vi "Align VI windows.vi"(4 "Keep on screen [T]":bool=TRUE, 5 "Align to":enum16{"FP", "BD"}(ring), 6 "Offset":cluster{"X":dbl, "Y":dbl}, 7 "Position [Center]":T2(ring)=enum."Center", 8 "error in":errorcluster, 10 "VI to Move Ref":refnum<vi>, 11 "Stationary VI Ref":refnum<vi>) -> (0 "error out":errorcluster)   [LabVIEW 2023]
doc: "Align two VI windows to center or one of the calling VIs corners. Offset is from calling VIs top left corner. \n\nYou can align to the stationary VI's front panel (default) or block diagram.\n\nWindow alignment can be on center or 12 other possible positions.\n\nThis VI operates on input error (input err merged with output error).\n\n'Keep on screen' (default=T) will automatically offset VI to Move window position to keep the top-left corner on the current monitor, to ensure that the title bar can be grabbed for moving the window."
uses:
  <userlib>/_OpenG.lib/appcontrol/appcontrol.llb/openg_application_control.lvlib
panel:
  out "New VI bounds":T1
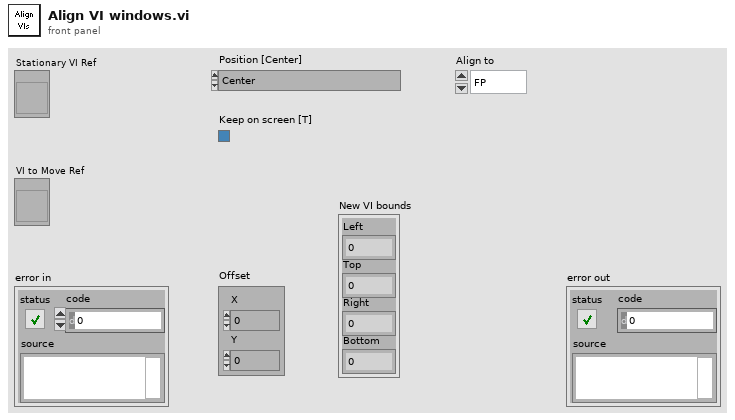
[diagram p1: front panel]
types:
  T1 = cluster{"Left":i16, "Top":i16, "Right":i16, "Bottom":i16}
  T2 = enum16{"Top Left", "Bottom Left", "Top Right", "Bottom Right", "Center", "Above Left", "Above Right", "Below Left", "Below Right", "Left Bottom", "Left Top", "Right Bottom", "Right Top", "Outside TL Corner", "Outside TR Corner", "Outside BL Corner", "Outside BR Corner"}
  T3 = enum16{"Top Left", "Bottom Left", "Top Right", "Bottom Right", "Center"}
  T4 = typedef "LVRectTypeDef.ctl" = cluster{"Left":i16, "Top":i16, "Right":i16, "Bottom":i16}
  T5 = typedef "x,y cluster_DBL.ctl" = cluster{"X":dbl, "Y":dbl}
  T6 = cluster{"left":i16, "top":i16, "right":i16, "bottom":i16}
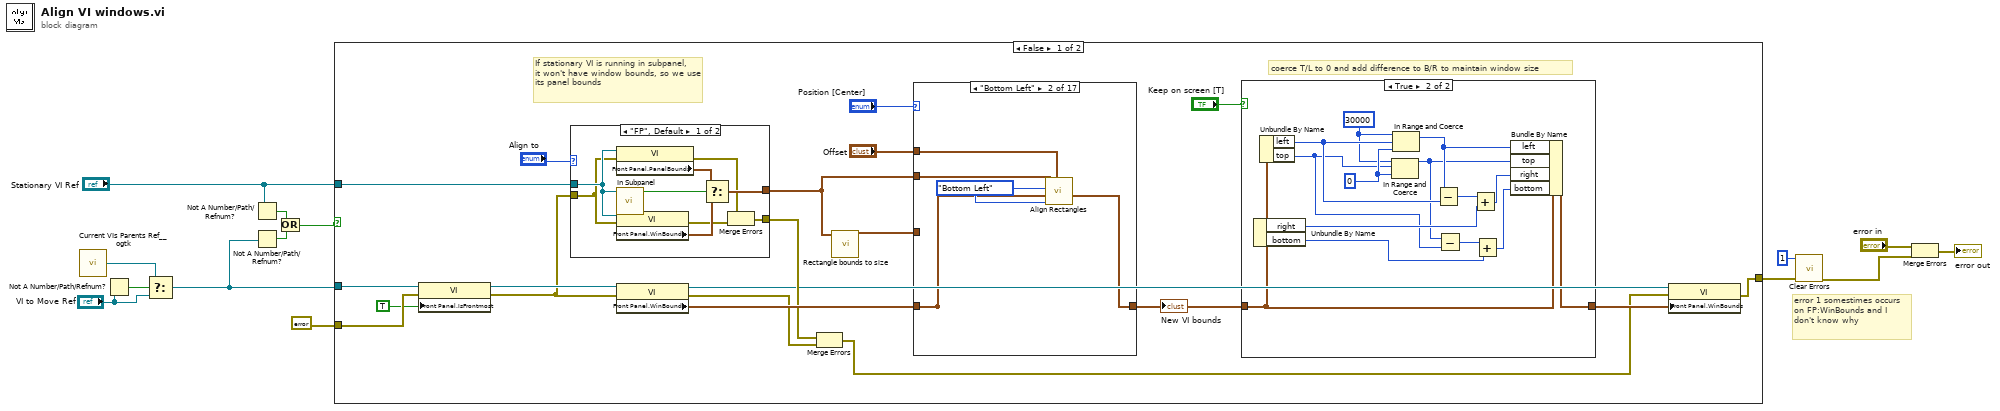
[diagram p0: block diagram]
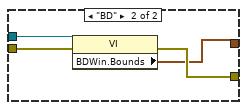
[diagram p3: hidden frame]
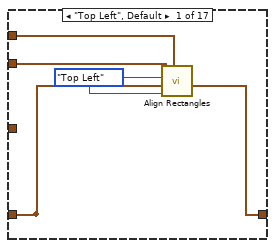
[diagram p4: hidden frame]
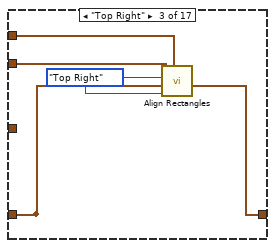
[diagram p5: hidden frame]
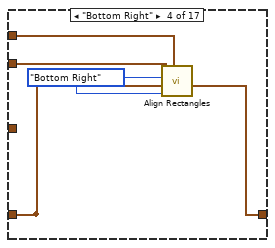
[diagram p6: hidden frame]
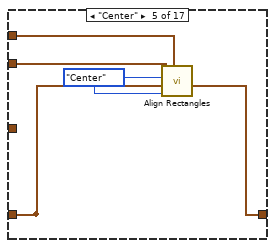
[diagram p7: hidden frame]
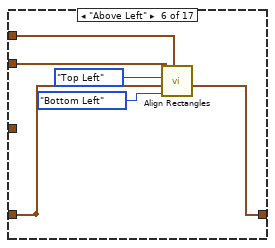
[diagram p8: hidden frame]
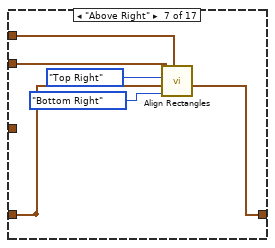
[diagram p9: hidden frame]
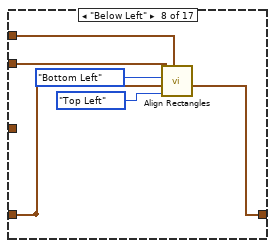
[diagram p10: hidden frame]
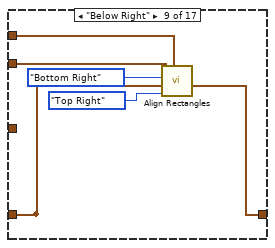
[diagram p11: hidden frame]
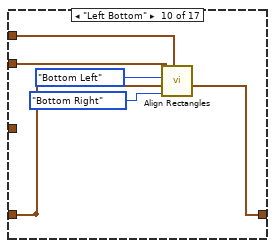
[diagram p12: hidden frame]
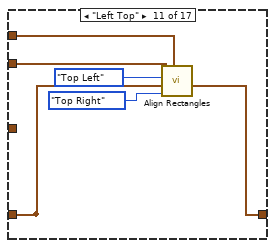
[diagram p13: hidden frame]
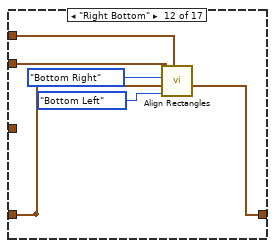
[diagram p14: hidden frame]
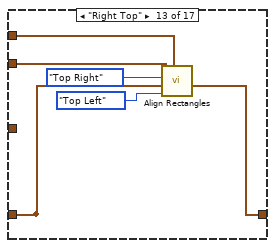
[diagram p15: hidden frame]
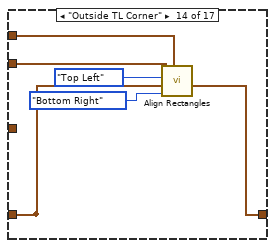
[diagram p16: hidden frame]
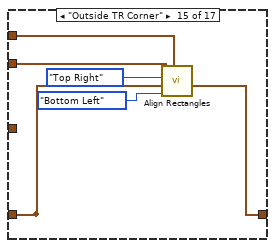
[diagram p17: hidden frame]
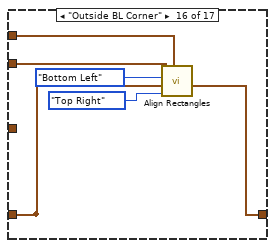
[diagram p18: hidden frame]
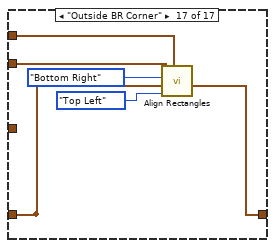
[diagram p19: hidden frame]
diagram:
  # "error 1 somestimes occurs on FP:WinBounds and I don't know why"
  n1 = call <userlib>:"Current VIs Parents Ref__ogtk.vi"() -> ("Calling VI's Reference"=w1:refnum<vi>)  [unwired: 2 in]
  n2 = Not A Number/Path/Refnum?(number/path/refnum="VI to Move Ref") -> (NaN/Path/Refnum?=w4:bool)
  n3 = Select(t=w1, s=w4, f="VI to Move Ref") -> (s? t:f=w2:refnum<vi>)
  n4 = Not A Number/Path/Refnum?(number/path/refnum="Stationary VI Ref") -> (NaN/Path/Refnum?=w14:bool)
  n5 = Not A Number/Path/Refnum?(number/path/refnum=w2) -> (NaN/Path/Refnum?=w13:bool)
  n6 = Or(x=w14, y=w13) -> (x .or. y?=w11:bool)
  n7 = case shown="False" w11 {
    tunnel: "Stationary VI Ref" -> [w29 _]
    tunnel: errorcluster {"status"=FALSE, "code"=0, "source"=""} ("error in (no error)") -> [w16 w159]
    tunnel: [w30 w159] -> w7
    tunnel: w2 -> [w19 _]
    frame False {
      # "coerce T/L to 0 and add difference to B/R to maintain window size"
      # "If stationary VI is running in subpanel, it won't have window bounds, so we use its panel bounds"
      n8 = property class="VI"(reference=w19, error in=w16, "Front Panel.IsFrontmost"=TRUE ("Front Panel Window:Is Frontmost")) -> (reference out=w18:refnum<vi>, error out=w17:errorcluster)
      n9 = case shown="\"FP\", Default" "Align to" {
        tunnel: w29 -> [w57 w61]
        tunnel: [w54 w58] -> w28
        tunnel: w17 -> [w53 w60]
        tunnel: [w50 w59] -> w26
        frame "FP", Default {
          n10 = property class="VI"(reference=w57, error in=w53) -> (error out=w51:errorcluster, "Front Panel.PanelBounds"=w56:T4)  [unwired: 1 out]
          n11 = call "In Subpanel.vi"("VI Ref"=w57) -> ("VI in SubPanel?"=w49:bool)  [unwired: 10 in]
          n12 = property class="VI"(reference=w57, error in=w53) -> (error out=w52:errorcluster, "Front Panel.WinBounds"=w55:T4)  [unwired: 1 out]
          n13 = Select(t=w56, s=w49, f=w55) -> (s? t:f=w54:T4)
          n14 = Merge Errors(w51, w52) -> (w50:errorcluster)
        }
        frame "BD" {
          n15 = property class="VI"(reference=w61, error in=w60) -> (error out=w59:errorcluster, "BDWin.Bounds"=w58:T4)  [unwired: 1 out]
        }
      }
      n16 = property class="VI"(reference=w18, error in=w17) -> (error out=w21:errorcluster, "Front Panel.WinBounds"=w27:T4)  [unwired: 1 out]
      n17 = Merge Errors(w26, w21) -> (w20:errorcluster)
      n18 = call "Rectangle bounds to size.vi"("bounds"=w28) -> ("size"=w32:T5)  [unwired: 6 in, 4 out]
      n19 = case shown="\"Bottom Left\"" "Position [Center]" {
        tunnel: w32 -> [_ _ _ _ _ _ _ _ _ _ _ _ _ _ _ _ _]
        tunnel: w28 -> [w63 w68 w73 w78 w83 w89 w95 w101 w107 w113 w119 w125 w131 w137 w143 w149 w155]
        tunnel: [w62 w67 w72 w77 w82 w88 w94 w100 w106 w112 w118 w124 w130 w136 w142 w148 w154] -> _
        tunnel: "Offset" -> [w65 w70 w75 w80 w85 w91 w97 w103 w109 w115 w121 w127 w133 w139 w145 w151 w157]
        tunnel: [w64 w69 w74 w79 w84 w90 w96 w102 w108 w114 w120 w126 w132 w138 w144 w150 w156] -> w24
        tunnel: w27 -> [w62 w67 w72 w77 w82 w88 w94 w100 w106 w112 w118 w124 w130 w136 w142 w148 w154]
        frame "Top Left", Default {
          w66 = T3."Top Left" ("Position 1 [Top-Left]")
          n20 = call "Align Rectangles.vi"("Offset"=w65, "Position 2 [Top-Left]"=w66, "rect 2"=w62, "Position 1 [Top-Left]"=w66, "rect 1"=w63) -> ("rect out"=w64:T6)  [unwired: 6 in]
        }
        frame "Bottom Left" {
          w71 = T3."Bottom Left" ("Position 1 [Top-Left]")
          n21 = call "Align Rectangles.vi"("Offset"=w70, "Position 2 [Top-Left]"=w71, "rect 2"=w67, "Position 1 [Top-Left]"=w71, "rect 1"=w68) -> ("rect out"=w69:T6)  [unwired: 6 in]
        }
        frame "Top Right" {
          w76 = T3."Top Right" ("Position 1 [Top-Left]")
          n22 = call "Align Rectangles.vi"("Offset"=w75, "Position 2 [Top-Left]"=w76, "rect 2"=w72, "Position 1 [Top-Left]"=w76, "rect 1"=w73) -> ("rect out"=w74:T6)  [unwired: 6 in]
        }
        frame "Bottom Right" {
          w81 = T3."Bottom Right" ("Position 1 [Top-Left]")
          n23 = call "Align Rectangles.vi"("Offset"=w80, "Position 2 [Top-Left]"=w81, "rect 2"=w77, "Position 1 [Top-Left]"=w81, "rect 1"=w78) -> ("rect out"=w79:T6)  [unwired: 6 in]
        }
        frame "Center" {
          w86 = T3."Center" ("Position 1 [Top-Left]")
          n24 = call "Align Rectangles.vi"("Offset"=w85, "Position 2 [Top-Left]"=w86, "rect 2"=w82, "Position 1 [Top-Left]"=w86, "rect 1"=w83) -> ("rect out"=w84:T6)  [unwired: 6 in]
        }
        frame "Above Left" {
          n25 = call "Align Rectangles.vi"("Offset"=w91, "Position 2 [Top-Left]"=T3."Bottom Left" ("Position 1 [Top-Left]"), "rect 2"=w88, "Position 1 [Top-Left]"=T3."Top Left", "rect 1"=w89) -> ("rect out"=w90:T6)  [unwired: 6 in]
        }
        frame "Above Right" {
          n26 = call "Align Rectangles.vi"("Offset"=w97, "Position 2 [Top-Left]"=T3."Bottom Right" ("Position 1 [Top-Left]"), "rect 2"=w94, "Position 1 [Top-Left]"=T3."Top Right", "rect 1"=w95) -> ("rect out"=w96:T6)  [unwired: 6 in]
        }
        frame "Below Left" {
          n27 = call "Align Rectangles.vi"("Offset"=w103, "Position 2 [Top-Left]"=T3."Top Left" ("Position 1 [Top-Left]"), "rect 2"=w100, "Position 1 [Top-Left]"=T3."Bottom Left", "rect 1"=w101) -> ("rect out"=w102:T6)  [unwired: 6 in]
        }
        frame "Below Right" {
          n28 = call "Align Rectangles.vi"("Offset"=w109, "Position 2 [Top-Left]"=T3."Top Right" ("Position 1 [Top-Left]"), "rect 2"=w106, "Position 1 [Top-Left]"=T3."Bottom Right", "rect 1"=w107) -> ("rect out"=w108:T6)  [unwired: 6 in]
        }
        frame "Left Bottom" {
          n29 = call "Align Rectangles.vi"("Offset"=w115, "Position 2 [Top-Left]"=T3."Bottom Right" ("Position 1 [Top-Left]"), "rect 2"=w112, "Position 1 [Top-Left]"=T3."Bottom Left", "rect 1"=w113) -> ("rect out"=w114:T6)  [unwired: 6 in]
        }
        frame "Left Top" {
          n30 = call "Align Rectangles.vi"("Offset"=w121, "Position 2 [Top-Left]"=T3."Top Right" ("Position 1 [Top-Left]"), "rect 2"=w118, "Position 1 [Top-Left]"=T3."Top Left", "rect 1"=w119) -> ("rect out"=w120:T6)  [unwired: 6 in]
        }
        frame "Right Bottom" {
          n31 = call "Align Rectangles.vi"("Offset"=w127, "Position 2 [Top-Left]"=T3."Bottom Left" ("Position 1 [Top-Left]"), "rect 2"=w124, "Position 1 [Top-Left]"=T3."Bottom Right", "rect 1"=w125) -> ("rect out"=w126:T6)  [unwired: 6 in]
        }
        frame "Right Top" {
          n32 = call "Align Rectangles.vi"("Offset"=w133, "Position 2 [Top-Left]"=T3."Top Left" ("Position 1 [Top-Left]"), "rect 2"=w130, "Position 1 [Top-Left]"=T3."Top Right", "rect 1"=w131) -> ("rect out"=w132:T6)  [unwired: 6 in]
        }
        frame "Outside TL Corner" {
          n33 = call "Align Rectangles.vi"("Offset"=w139, "Position 2 [Top-Left]"=T3."Bottom Right" ("Position 1 [Top-Left]"), "rect 2"=w136, "Position 1 [Top-Left]"=T3."Top Left", "rect 1"=w137) -> ("rect out"=w138:T6)  [unwired: 6 in]
        }
        frame "Outside TR Corner" {
          n34 = call "Align Rectangles.vi"("Offset"=w145, "Position 2 [Top-Left]"=T3."Bottom Left" ("Position 1 [Top-Left]"), "rect 2"=w142, "Position 1 [Top-Left]"=T3."Top Right", "rect 1"=w143) -> ("rect out"=w144:T6)  [unwired: 6 in]
        }
        frame "Outside BL Corner" {
          n35 = call "Align Rectangles.vi"("Offset"=w151, "Position 2 [Top-Left]"=T3."Top Right" ("Position 1 [Top-Left]"), "rect 2"=w148, "Position 1 [Top-Left]"=T3."Bottom Left", "rect 1"=w149) -> ("rect out"=w150:T6)  [unwired: 6 in]
        }
        frame "Outside BR Corner" {
          n36 = call "Align Rectangles.vi"("Offset"=w157, "Position 2 [Top-Left]"=T3."Top Left" ("Position 1 [Top-Left]"), "rect 2"=w154, "Position 1 [Top-Left]"=T3."Bottom Right", "rect 1"=w155) -> ("rect out"=w156:T6)  [unwired: 6 in]
        }
      }
      "New VI bounds" <- w24
      n37 = case shown="True" "Keep on screen [T]" {
        tunnel: w24 -> [w34 w44]
        tunnel: [w34 w47] -> w22
        frame False {
        }
        frame True {
          w35 = 30000 ("upper limit")
          w48 = 0
          n38 = Unbundle By Name(w44) -> ("right"=w42:i16, "bottom"=w36:i16)
          n39 = Unbundle By Name(w44) -> ("left"=w45:i16, "top"=w37:i16)
          n40 = In Range and Coerce(upper limit=w35, x=w37, lower limit=w48) -> (coerced(x)=w39:i32)  [unwired: 1 out]
          n41 = In Range and Coerce(upper limit=w35, x=w45, lower limit=w48) -> (coerced(x)=w46:i32)  [unwired: 1 out]
          n42 = Subtract(x=w46, y=w45) -> (x-y=w43:i32)
          n43 = Subtract(x=w39, y=w37) -> (x-y=w40:i32)
          n44 = Add(x=w43, y=w42) -> (x+y=w41:i32)
          n45 = Add(x=w40, y=w36) -> (x+y=w38:i32)
          n46 = Bundle By Name(cluster=w44, "left"=w46, "top"=w39, "right"=w41, "bottom"=w38) -> (w47:T6)
        }
      }
      n47 = property class="VI"(reference=w18, error in=w20, "Front Panel.WinBounds"=w22) -> (error out=w30:errorcluster)  [unwired: 1 out]
    }
    frame True {
    }
  }
  n48 = call <vilib>:"Clear Errors.vi"("error in (no error)"=w7, "specific error code to clear (0: all)"=1) -> ("error out"=w6:errorcluster)  [unwired: 4 in, 1 out]
  n49 = Merge Errors("error in", w6) -> (→"error out":errorcluster)
